vi "Launch Root Model.vi"(8 "error in (no error)":errorcluster, 11 "IViewModel In":refnum<class "IViewModel.lvclass">) -> (0 "error out":errorcluster, 3 "IViewModel Out":refnum<class "IViewModel.lvclass">)   [LabVIEW 2017, in "IViewModel.lvlib" / "IViewModel.lvclass"]
doc: "<License>\nCopyright © 2017 Composed Systems, LLC | All rights reserved\nwww.composed.io\n\nAuthor: Ethan Stern <ethan.stern@composed.io>\n\nThis software is provided \"AS IS\" WITHOUT WARRANTIES, either express or implied, AND IS FOR EDUCATIONAL PURPOSES ONLY.\n</License>"
uses:
  IViewModel.lvclass
  C:/Program Files (x86)/National Instruments/LabVIEW 2017/vi.lib/ActorFramework/Actor/Actor.lvclass
  C:/Git/mva-framework/Framework/IObserver/IObserver/IObserver.lvclass
  IMediator/IMediator Messages/Publish Msg/Publish Msg.lvclass
  C:/Git/mva-framework/Framework/AbstractMessages/PreAddressedMsg/PreAddressedMsg.lvclass
  IMediator/IMediator Messages/Subscribe Msg/Subscribe Msg.lvclass
  IMediator/IMediator Messages/Unsubscribe Msg/Unsubscribe Msg.lvclass
  IMediator/IMediator Messages/Lock Publication Msg/Lock Publication Msg.lvclass
  IMediator/IMediator Messages/Unlock Publication Msg/Unlock Publication Msg.lvclass
  IViewModel.lvclass/IViewModel.ctl
  AbstractMessages/PreAddressedMsg/PreAddressedMsg.lvclass/PreAddressedMsg.ctl
  IModel/IModel/IModel.lvclass/IModel.ctl
  IObserver/IObserver/IObserver.lvclass/IObserver.ctl
  IMediator/IMediator/IMediator.lvclass
  IModel/IModel/IModel.lvclass
  <vilib>/ActorFramework/Actor/Actor.lvclass
  AbstractMessages/PreAddressedMsg/PreAddressedMsg.lvclass
  IObserver/IObserver/IObserver.lvclass
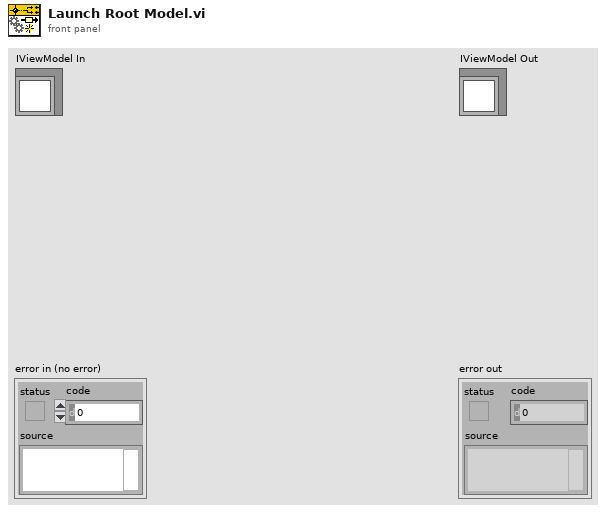
[diagram p1: front panel]
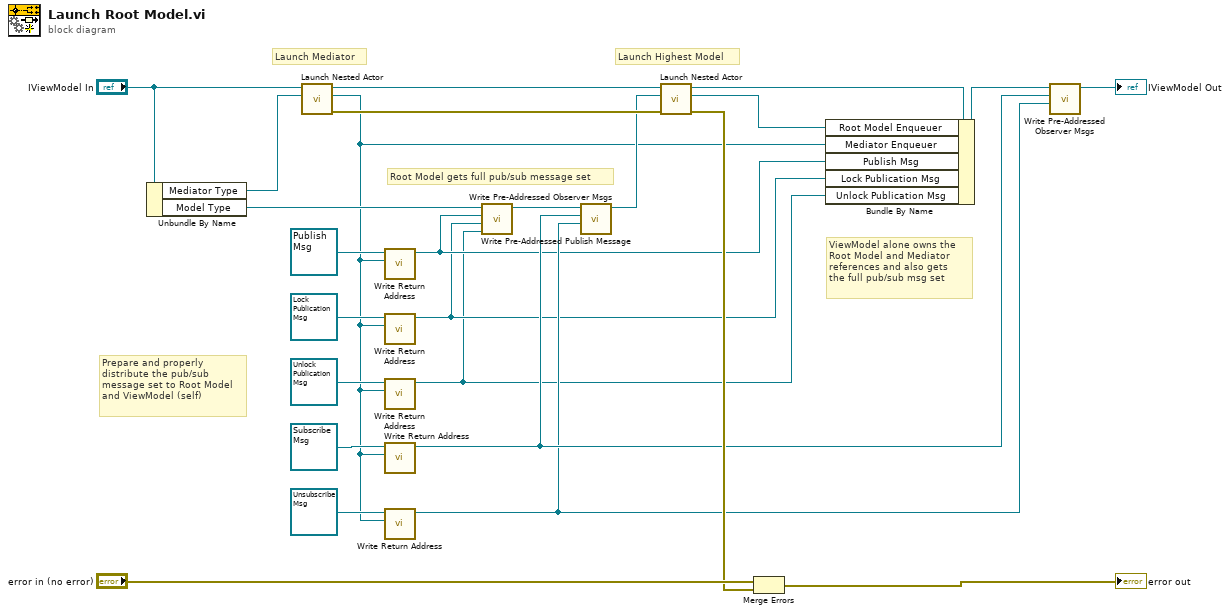
[diagram p0: block diagram]
diagram:
  # "Root Model gets full pub/sub message set"
  # "Prepare and properly\ndistribute the pub/sub\nmessage set to Root Model\nand ViewModel (self)"
  # "Launch Highest Model"
  # "Launch Mediator"
  # "ViewModel alone owns the\nRoot Model and Mediator\nreferences and also gets\nthe full pub/sub msg set"
  n1 = Unbundle By Name("IViewModel In") -> ("Mediator Type"=w21:refnum<class "IMediator.lvclass">, "Model Type"=w20:refnum<class "IModel.lvclass">)
  n2 = call <vilib>:"Launch Nested Actor.vi"("Nested Actor"=w21, "Caller Actor in"="IViewModel In") -> ("error out"=w16:errorcluster, "Nested Actor's Enqueuer"=w1:refnum<class "Message Enqueuer.lvclass">, "Caller Actor out"=w22:refnum<class "IViewModel.lvclass">)  [unwired: 7 in]
  n3 = call "Write Return Address.vi"("Return Address"=w1, "PreAddressedMsg in"=refnum<class "Publish Msg.lvclass"> refnum ("IMediator.lvlib:Publish Msg.lvclass")) -> ("PreAddressedMsg out"=w6:refnum<class "Publish Msg.lvclass">)  [unwired: 9 in]
  n4 = call "Write Return Address.vi"("Return Address"=w1, "PreAddressedMsg in"=refnum<class "Lock Publication Msg.lvclass"> refnum ("Lock Publication Msg")) -> ("PreAddressedMsg out"=w3:refnum<class "Lock Publication Msg.lvclass">)  [unwired: 9 in]
  n5 = call "Write Return Address.vi"("Return Address"=w1, "PreAddressedMsg in"=refnum<class "Unlock Publication Msg.lvclass"> refnum ("Unlock Publication Msg")) -> ("PreAddressedMsg out"=w2:refnum<class "Unlock Publication Msg.lvclass">)  [unwired: 9 in]
  n6 = call "Write Return Address.vi"("Return Address"=w1, "PreAddressedMsg in"=refnum<class "Subscribe Msg.lvclass"> refnum ("IMediator.lvlib:Subscribe Msg.lvclass")) -> ("PreAddressedMsg out"=w8:refnum<class "Subscribe Msg.lvclass">)  [unwired: 9 in]
  n7 = call "Write Return Address.vi"("Return Address"=w1, "PreAddressedMsg in"=refnum<class "Unsubscribe Msg.lvclass"> refnum ("IMediator.lvlib:Unsubscribe Msg.lvclass")) -> ("PreAddressedMsg out"=w7:refnum<class "Unsubscribe Msg.lvclass">)  [unwired: 9 in]
  n8 = call "Write Pre-Addressed Publish Message.vi"("Pre-Addressed Unlock Publication Msg"=w2, "Pre-Addressed Lock Publication Msg"=w3, "Pre-Addressed Publish Msg"=w6, "IModel in"=w20) -> ("IModel out"=w12:refnum<class "IModel.lvclass">)  [unwired: 7 in]
  n9 = call "Write Pre-Addressed Observer Msgs.vi"("Pre-Addressed Unsubscribe Msg"=w7, "Pre-Addressed Subscribe Msg"=w8, "IObserver In"=w12) -> ("IObserver Out"=w11:refnum<class "IModel.lvclass">)  [unwired: 8 in]
  n10 = call <vilib>:"Launch Nested Actor.vi"("error in (no error)"=w16, "Nested Actor"=w11, "Caller Actor in"=w22) -> ("error out"=w14:errorcluster, "Nested Actor's Enqueuer"=w17:refnum<class "Message Enqueuer.lvclass">, "Caller Actor out"=w19:refnum<class "IViewModel.lvclass">)  [unwired: 6 in]
  n11 = Merge Errors("error in (no error)", w14) -> (→"error out":errorcluster)
  n12 = Bundle By Name(cluster=w19, "Root Model Enqueuer"=w17, "Mediator Enqueuer"=w1, "Publish Msg"=w6, "Lock Publication Msg"=w3, "Unlock Publication Msg"=w2) -> (w18:refnum<class "IViewModel.lvclass">)
  n13 = call "Write Pre-Addressed Observer Msgs.vi"("Pre-Addressed Unsubscribe Msg"=w7, "Pre-Addressed Subscribe Msg"=w8, "IObserver In"=w18) -> ("IObserver Out"=→"IViewModel Out":refnum<class "IViewModel.lvclass">)  [unwired: 8 in]
